vi "Write Sub Panel coin.vi"(8 "error in (no error)":errorcluster, 10 "Sub Panel coin":refnum<vi>, 11 "MXN actor in":refnum<class "MXN actor.lvclass">) -> (0 "error out":errorcluster, 3 "MXN actor out":refnum<class "MXN actor.lvclass">)   [LabVIEW 2020, in "MXN actor.lvlib" / "MXN actor.lvclass"]
uses:
  MXN actor.lvclass
  MXN actor.lvclass/MXN actor.ctl
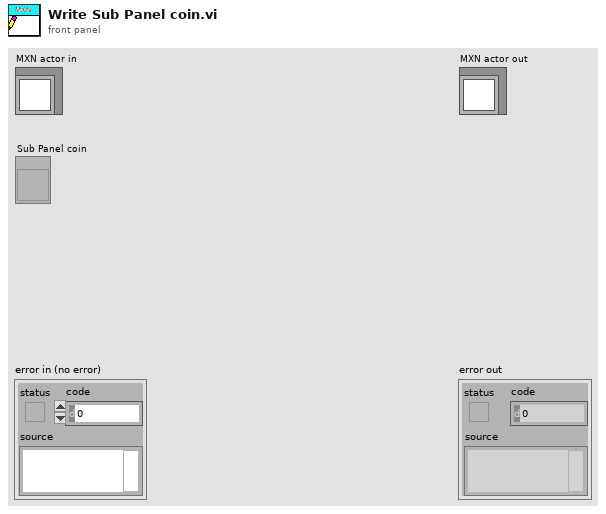
[diagram p1: front panel]
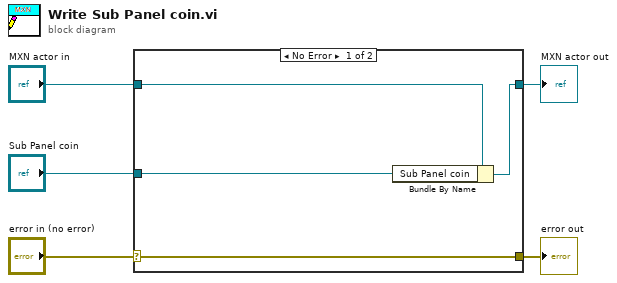
[diagram p0: block diagram]
diagram:
  n1 = case shown="No Error" "error in (no error)" {
    selector: "error in (no error)" -> [w9 w10]
    tunnel: [w9 w10] -> w4
    tunnel: [w7 w11] -> w2
    tunnel: "MXN actor in" -> [w8 w11]
    tunnel: "Sub Panel coin" -> [w6 _]
    frame No Error {
      n2 = Bundle By Name(cluster=w8, "Sub Panel coin"=w6) -> (w7:refnum<class "MXN actor.lvclass">)
    }
    frame Error {
    }
  }
  "error out" <- w4
  "MXN actor out" <- w2
